vi "Сумматор 4.vi"(2 "?":bool, 3 "B":T2, 4 "A":T1) -> (0 "Summ":T1, 1 "?":bool)   [LabVIEW 2017]
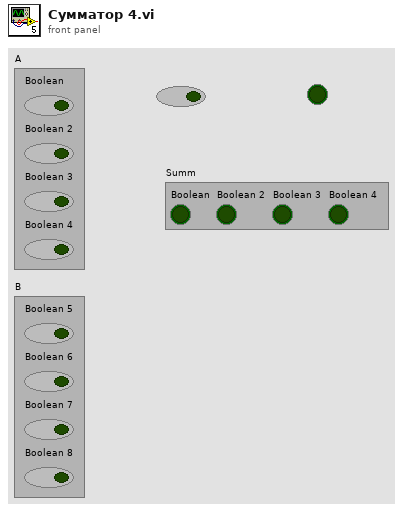
[diagram p1: front panel]
types:
  T1 = cluster{"Boolean":bool, "Boolean 2":bool, "Boolean 3":bool, "Boolean 4":bool}
  T2 = cluster{"Boolean 5":bool, "Boolean 6":bool, "Boolean 7":bool, "Boolean 8":bool}
  T3 = cluster{"Si":bool, "Si":bool, "Si":bool, "Si":bool}
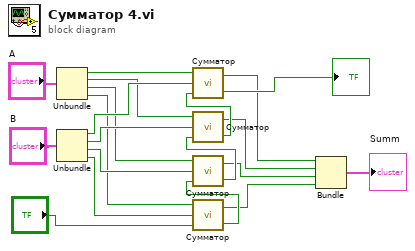
[diagram p0: block diagram]
diagram:
  n1 = Unbundle("A") -> ("Boolean"=w11:bool, "Boolean 2"=w12:bool, "Boolean 3"=w13:bool, "Boolean 4"=w14:bool)
  n2 = Unbundle("B") -> ("Boolean 5"=w15:bool, "Boolean 6"=w16:bool, "Boolean 7"=w17:bool, "Boolean 8"=w18:bool)
  n3 = call "Сумматор.vi"("i-1"="?", "B"=w18, "A"=w14) -> ("Ci"=w10:bool, "Si"=w3:bool)
  n4 = call "Сумматор.vi"("i-1"=w10, "B"=w17, "A"=w13) -> ("Ci"=w9:bool, "Si"=w2:bool)
  n5 = call "Сумматор.vi"("i-1"=w9, "B"=w16, "A"=w12) -> ("Ci"=w8:bool, "Si"=w4:bool)
  n6 = call "Сумматор.vi"("i-1"=w8, "B"=w15, "A"=w11) -> ("Ci"=→"?":bool, "Si"=w5:bool)
  n7 = Bundle("Si"=w5, "Si"=w4, "Si"=w2, "Si"=w3) -> (→"Summ":T3)  [unwired: 1 in]
